vi "Save Load FP.vi"(7 "Menu":enum16{"Save", "Load"}(ring), 8 "error in":errorcluster caption="에러 입력(에러 없음)", 11 "VI 참조 번호":refnum<vi>) -> (0 "error out":errorcluster caption="에러 출력", 3 "VI 참조 번호 out":refnum<vi>)   [LabVIEW 2020]
uses:
  <vilib>/Utility/sysdir.llb/System Directory Type.ctl
  Controls/Cmd_File path.ctl
  Controls/Cmd_File Type.ctl
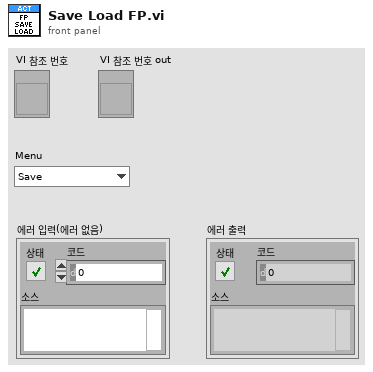
[diagram p1: front panel]
types:
  T1 = typedef "Cmd_File Type.ctl" = enum16{"엑셀", "엑셀(2003)", "텍스트", "설정", "2진", "VI", "CSV", "LOG", "폴더"}
  T2 = typedef "Cmd_File path.ctl" = enum16{"에러로그", "데이터파일경로", "성적서원본", "지난성적서", "Data Files", "경로생성", "Updater", "Template", "설정파일경로", "FTP Upload", "Update 경로", "어플리케이션"}
  T3 = enum16{"open", "replace", "create", "open or create", "replace or create", "replace or create with confirmation"}
  T4 = typedef "System Directory Type.ctl" = i32
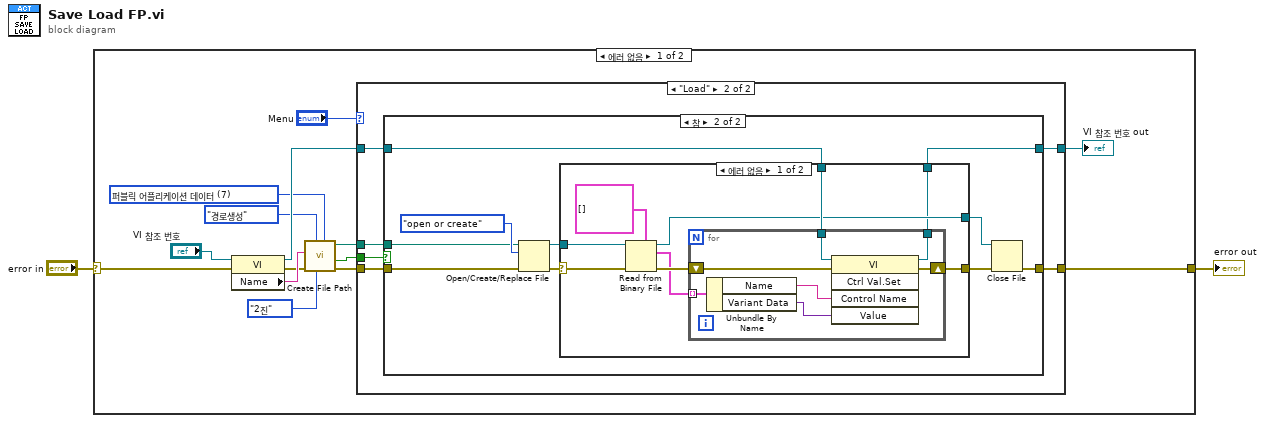
[diagram p0: block diagram]
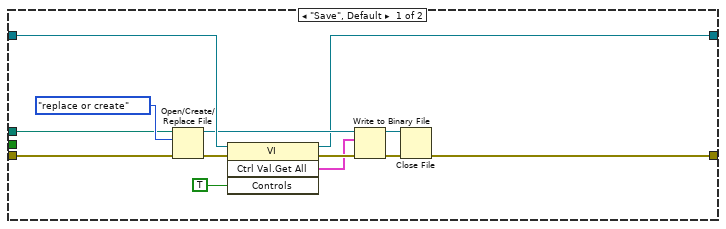
[diagram p2: hidden frame]
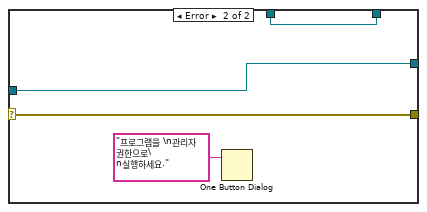
[diagram p4: hidden frame]
diagram:
  n1 = case shown="에러 없음" "error in" {
    selector: "error in" -> [w16 w68]
    tunnel: [w13 w68] -> w1
    frame No Error {
      w9 = T4 7 items=["사용자 홈"=0, "사용자 데스크탑"=1, "사용자 문서"=2, "사용자 어플리케이션 데이터"=3, "사용자 환경"=4, "사용자 임시"=5, "퍼블릭 문서"=6, "퍼블릭 어플리케이션 데이터"=7, "퍼블릭 환경"=8, "퍼블릭 캐시"=13, "시스템 코어 라이브러리"=9, "시스템 설치된 라이브러리"=10, "어플리케이션 파일"=11, "부팅 볼륨 루트"=12] ("system directory type")
      n2 = property class="VI"(reference="VI 참조 번호", error in=w16) -> (reference out=w14:refnum<vi>, error out=w5:errorcluster, "Name"=w10:string)
      n3 = call "Create File Path.vi"("system directory type"=w9, "파일타입"=Cmd_File_Type."2진", "항목"=Cmd_File_path."경로생성", "에러 입력"=w5, "문자열 in"=w10) -> ("error out"=w4:errorcluster, "파일존재?"=w6:bool, "파일경로"=w7:path)  [unwired: 3 in, 1 out]
      n4 = case shown="\"Load\"" "Menu" {
        tunnel: w14 -> [w29 w34]
        tunnel: w4 -> [w18 w35]
        tunnel: [w22 w33] -> w13
        tunnel: [w19 w32] -> w11
        tunnel: w7 -> [w17 w30]
        tunnel: w6 -> [_ w31]
        frame "Save", Default {
          n5 = Open/Create/Replace File(file path (use dialog)=w17, error in=w18, operation (0:open)=T3."replace or create" ("동작(0:open)")) -> (refnum out=w24:refnum<file>, error out=w20:errorcluster)  [unwired: 3 in, 1 out]
          n6 = invoke class="VI" method="Ctrl Val.Get All"(reference=w29, error in=w20, "Controls"=TRUE ("컨트롤")) -> (reference out=w19:refnum<vi>, error out=w26:errorcluster, "Get All Control Values Variant"=w21:cluster{"Name":string, "Variant Data":variant}[])  [unwired: 1 in, 1 out]
          n7 = Write to Binary File(file (use dialog)=w24, data=w21, error in=w26) -> (refnum out=w23:refnum<file>, error out=w25:errorcluster)  [unwired: 3 in, 1 out]
          n8 = Close File(refnum=w23, error in=w25) -> (error out=w22:errorcluster)  [unwired: 1 out]
        }
        frame "Load" {
          n9 = case shown="참" w31 {
            tunnel: w30 -> [_ w46]
            tunnel: w35 -> [w37 w45]
            tunnel: w34 -> [w36 w41]
            tunnel: [w37 w44] -> w33
            tunnel: [w36 w39] -> w32
            frame False {
            }
            frame True {
              n10 = Open/Create/Replace File(file path (use dialog)=w46, error in=w45, operation (0:open)=T3."open or create" ("동작(0:open)")) -> (refnum out=w42:refnum<file>, error out=w43:errorcluster)  [unwired: 3 in, 1 out]
              n11 = case shown="에러 없음" w43 {
                selector: w43 -> [w55 w64]
                tunnel: w42 -> [w54 w65]
                tunnel: w41 -> [w52 w66]
                tunnel: [w50 w65] -> w40
                tunnel: [w49 w66] -> w39
                tunnel: [w48 w64] -> w38
                frame No Error {
                  n12 = Read from Binary File(5:cluster{"Name":string, "Variant Data":variant}[] [] ("컨트롤 값:모두 얻기"), 8:w55, 11:w54) -> (0:w53:errorcluster, 2:w51:cluster{"Name":string, "Variant Data":variant}[], 3:w50:refnum<file>)  [unwired: 3 in, 1 out]
                  n13 = for {
                    tunnel: w52 -> [w62]
                    tunnel: w51 -> [w63] mode=indexing
                    tunnel: [w58] -> w49
                    shift-right: [w57] -> w48
                    shift-left: w53 -> [w59]
                    n14 = Unbundle By Name(w63) -> ("Name"=w61:string, "Variant Data"=w60:variant)
                    n15 = invoke class="VI" method="Ctrl Val.Set"(reference=w62, error in=w59, "Control Name"=w61, "Value"=w60) -> (reference out=w58:refnum<vi>, error out=w57:errorcluster)  [unwired: 1 in, 3 out]
                  }
                }
                frame Error {
                  n16 = One Button Dialog(message="프로그램을 \n관리자 권한으로\n실행하세요." ("메시지")) -> ()  [unwired: 1 in, 1 out]
                }
              }
              n17 = Close File(refnum=w40, error in=w38) -> (error out=w44:errorcluster)  [unwired: 1 out]
            }
          }
        }
      }
      "VI 참조 번호 out" <- w11
    }
    frame Error {
    }
  }
  "error out" <- w1
